vi "SetStatusRegisterFormat.vi"(8 "Error In":errorcluster, 10 "Status Register Format":T1, 11 "Keithley 6482 In":refnum<visa-resource-name>) -> (0 "Error Out":errorcluster, 3 "Keithley 6482 Out":refnum<visa-resource-name>)   [LabVIEW 2012, in "Keithley-6482.lvlib"]
uses:
  Keithley-6482.lvlib
  Controls/StatusRegisterFormat.ctl
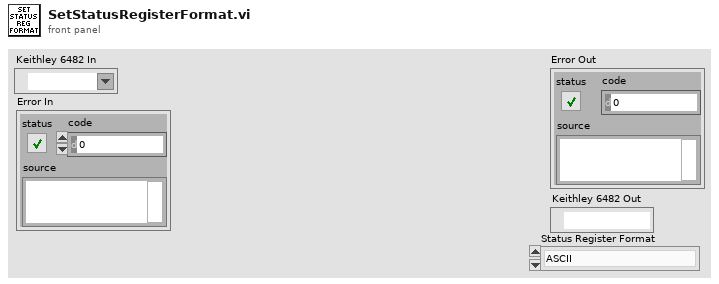
[diagram p1: front panel]
types:
  T1 = typedef "Keithley-6482.lvlib/StatusRegisterFormat.ctl" = enum16{"ASCII", "Hexadecimal", "Octal", "Binary"}
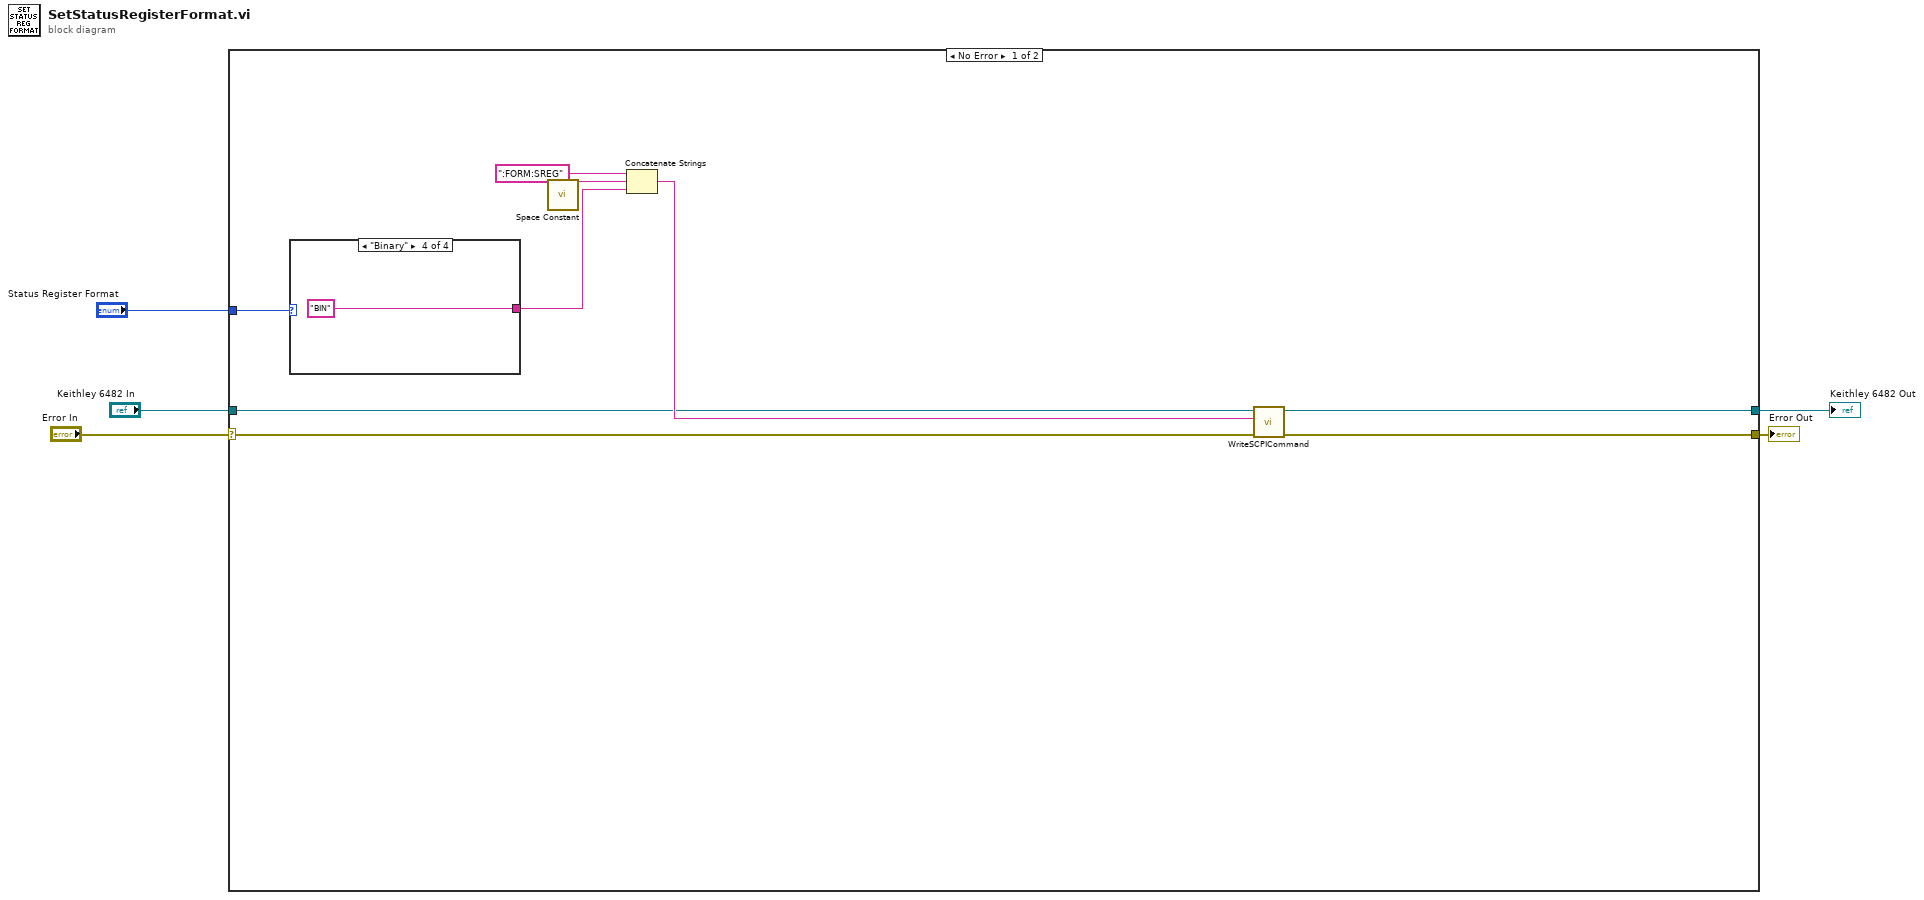
[diagram p0: block diagram]
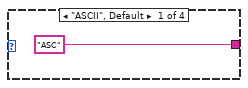
[diagram p2: hidden frame]
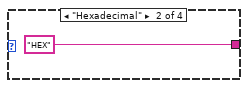
[diagram p3: hidden frame]
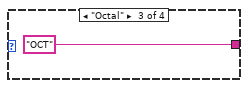
[diagram p4: hidden frame]
diagram:
  n1 = case shown="No Error" "Error In" {
    selector: "Error In" -> [w8 w19]
    tunnel: "Keithley 6482 In" -> [w6 w20]
    tunnel: [w9 w19] -> w3
    tunnel: [w10 w20] -> w2
    tunnel: "Status Register Format" -> [w12 _]
    frame No Error {
      n2 = case shown="\"Binary\"" w12 {
        tunnel: ["ASC" "HEX" "OCT" "BIN"] -> w11
        frame "ASCII", Default {
        }
        frame "Hexadecimal" {
        }
        frame "Octal" {
        }
        frame "Binary" {
        }
      }
      n3 = call <vilib>:"Space Constant.vi"() -> ("String"=w13:string)
      n4 = Concatenate Strings(":FORM:SREG", w13, w11) -> (w7:string)
      n5 = call "WriteSCPICommand.vi"("Error In"=w8, "SCPI Command"=w7, "Keithley 6482 In"=w6) -> ("Error Out"=w9:errorcluster, "Keithley 6482 Out"=w10:refnum<visa-resource-name>)  [unwired: 7 in]
    }
    frame Error {
    }
  }
  "Error Out" <- w3
  "Keithley 6482 Out" <- w2
